vi "Using_Formula_Node.vi"() -> ()   [LabVIEW 2017, in "Examples.lvlib"]
uses:
  Examples.lvlib
panel:
  out "Waveform Chart":dbl[][](graph)
  in  "b":dbl
  in  "m":dbl
  out "y":dbl
  in  "m":dbl
  in  "x":dbl
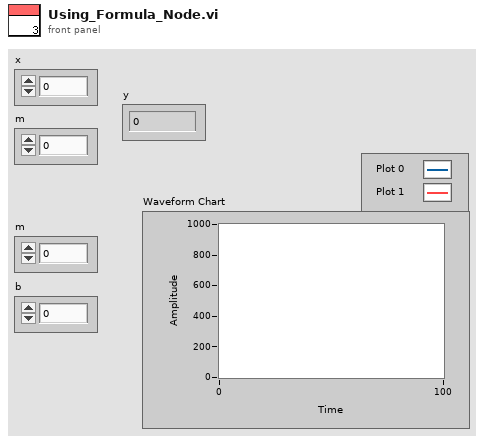
[diagram p1: front panel]
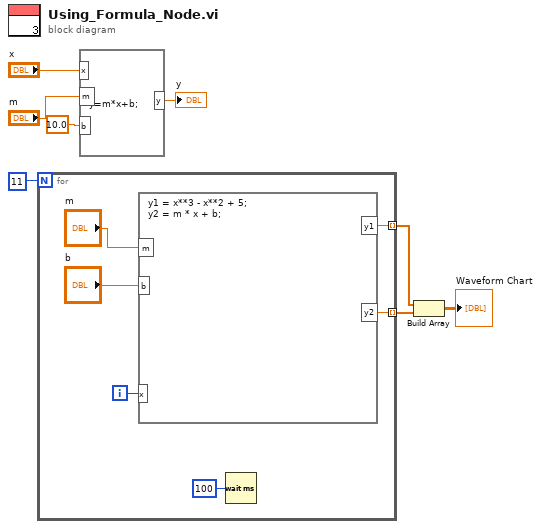
[diagram p0: block diagram]
diagram:
  n1 = for {
    N: 11 -> [_]
    tunnel: [w13] -> w3 mode=indexing
    tunnel: [w12] -> w2 mode=indexing
    i -> [w14]
    n2 = formula code="y1 = x**3 - x**2 + 5; \ny2 = m * x + b;"("m"="m", "b"="b", "x"=w14) -> ("y1"=w13:dbl, "y2"=w12:dbl)
    n3 = Wait (ms)(milliseconds to wait=u32 100) -> ()  [unwired: 1 out]
  }
  n4 = formula code="y=m*x+b;"("x"="x", "m"="m", "b"=10.0 ("input variable")) -> ("y"=→"y":dbl)
  n5 = Build Array(w3, w2) -> (→"Waveform Chart":dbl[][])
